vi "Read Write Unit Abbreviations.vi"(0 "Recommended In":T1(array[cluster]), 2 "ServerPath":path, 11 "Error In":errorcluster) -> (4 "Recommended Out":T1(array[cluster]), 8 "[Unit Abbr.s]":string[](array[string]), 10 "[Units]":string[](array[string]), 15 "Error Out":errorcluster)   [LabVIEW 2013]
uses:
  <vilib>/Utility/config.llb/Write Key (String).vi
  <vilib>/Utility/config.llb/Read Key (String).vi
  <vilib>/Utility/config.llb/NI_LVConfig.lvlib
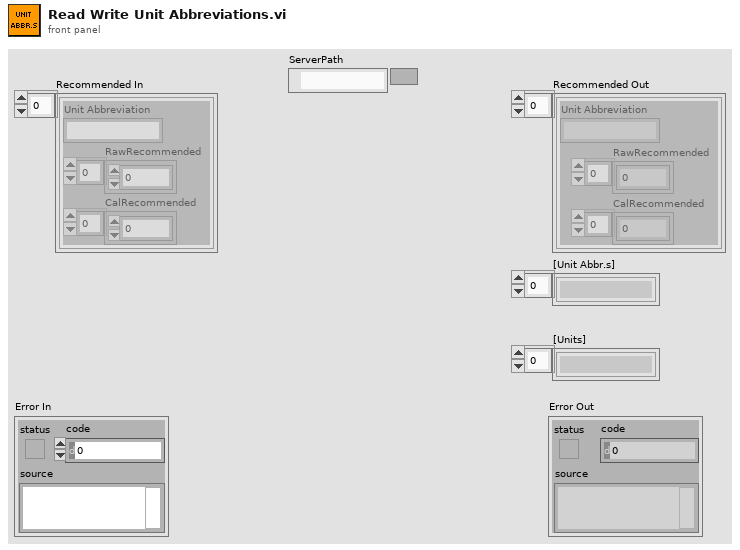
[diagram p1: front panel]
types:
  T1 = cluster{"Unit Abbreviation":string, "RawRecommended":dbl[], "CalRecommended":dbl[]}[]
  T2 = typedef "NI_LVConfig.lvlib/Config Data RefNum.ctl" = refnum<k1>
  T3 = cluster{"Unit Abbreviation":string, "RawRecommended":dbl[], "CalRecommended":dbl[]}
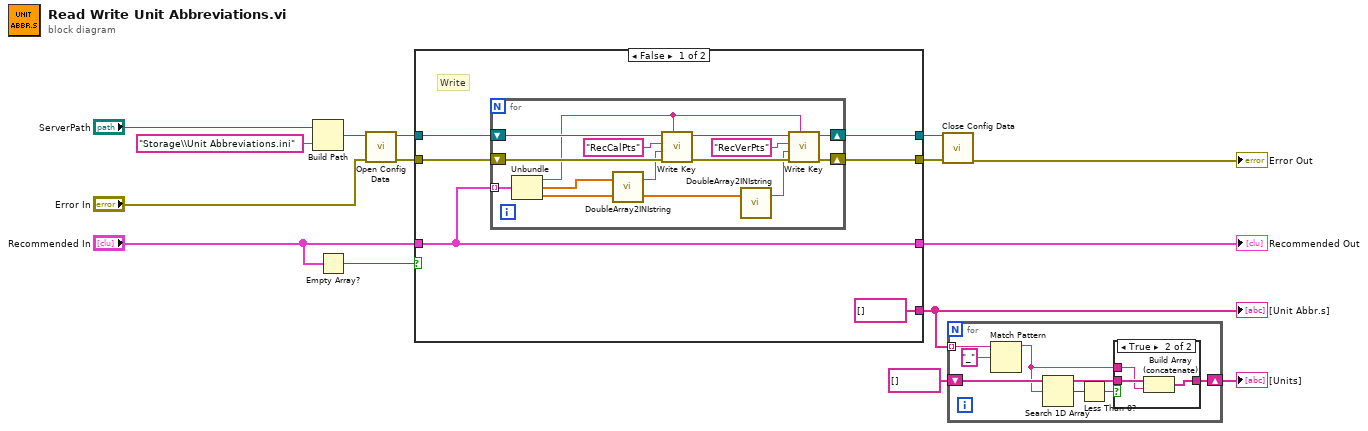
[diagram p0: block diagram]
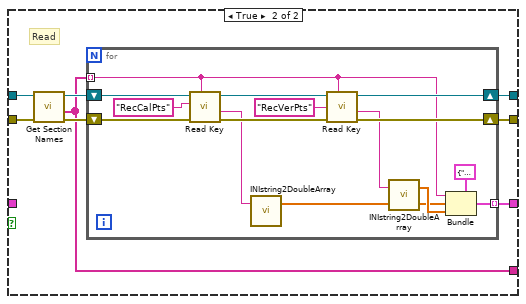
[diagram p3: hidden frame]
diagram:
  n1 = Build Path(base path="ServerPath", name or relative path="Storage\\Unit Abbreviations.ini") -> (appended path=w11:path)
  n2 = Empty Array?(array="Recommended In") -> (empty?=w13:bool)
  n3 = call <vilib>:"Open Config Data.vi"("error in (no error)"="Error In", "configuration file path"=w11) -> ("error out"=w8:errorcluster, "refnum"=w9:T2)  [unwired: 7 in, 1 out]
  n4 = case shown="False" w13 {
    tunnel: "Recommended In" -> [w17 _]
    tunnel: w9 -> [w21 w43]
    tunnel: w8 -> [w20 w42]
    tunnel: [w19 w39] -> w7
    tunnel: [w18 w38] -> w6
    tunnel: [w17 w37] -> w4
    tunnel: [string[] [] ("section names") w36] -> w3
    frame False {
      # "Write"
      n5 = for {
        shift-right: [w29] -> w19
        shift-left: w21 -> [w35]
        shift-right: [w30] -> w18
        shift-left: w20 -> [w34]
        tunnel: w17 -> [w33] mode=indexing
        n6 = Unbundle(w33) -> ("Unit Abbreviation"=w28:string, "RawRecommended"=w25:dbl[], "CalRecommended"=w24:dbl[])
        n7 = call "DoubleArray2INIstring.vi"("Array"=w25) -> ("String"=w22:string)  [unwired: 6 in]
        n8 = call-poly <vilib>:"Write Key.vi"("section"=w28, "error in (no error)"=w34, "value"=w22, "key"="RecCalPts", "refnum"=w35) -> ("error out"=w31:errorcluster, "refnum out"=w32:T2)  [unwired: 4 in, 1 out]
        n9 = call "DoubleArray2INIstring.vi"("Array"=w24) -> ("String"=w23:string)  [unwired: 6 in]
        n10 = call-poly <vilib>:"Write Key.vi"("section"=w28, "error in (no error)"=w31, "value"=w23, "key"="RecVerPts", "refnum"=w32) -> ("error out"=w30:errorcluster, "refnum out"=w29:T2)  [unwired: 4 in, 1 out]
      }
    }
    frame True {
      # "Read"
      n11 = call <vilib>:"Get Section Names.vi"("error in (no error)"=w42, "refnum"=w43) -> ("error out"=w40:errorcluster, "section names"=w36:string[], "refnum out"=w41:T2)  [unwired: 7 in]
      n12 = for {
        shift-right: [w56] -> w39
        shift-left: w41 -> [w58]
        shift-right: [w55] -> w38
        shift-left: w40 -> [w53]
        tunnel: w36 -> [w47] mode=indexing
        tunnel: [w44] -> w37 mode=indexing
        n13 = call-poly <vilib>:"Read Key.vi"("section"=w47, "error in (no error)"=w53, "key"="RecCalPts", "refnum"=w58) -> ("error out"=w54:errorcluster, "value"=w50:string, "refnum out"=w57:T2)  [unwired: 4 in, 1 out]
        n14 = call "INIstring2DoubleArray.vi"("String"=w50) -> ("Array"=w45:dbl[])  [unwired: 6 in]
        n15 = call-poly <vilib>:"Read Key.vi"("section"=w47, "error in (no error)"=w54, "key"="RecVerPts", "refnum"=w57) -> ("error out"=w55:errorcluster, "value"=w49:string, "refnum out"=w56:T2)  [unwired: 4 in, 1 out]
        n16 = call "INIstring2DoubleArray.vi"("String"=w49) -> ("Array"=w46:dbl[])  [unwired: 6 in]
        n17 = Bundle(cluster=T3 {"Unit Abbreviation"="", "RawRecommended"=[], "CalRecommended"=[]}, "Unit Abbreviation"=w47, "RawRecommended"=w45, "CalRecommended"=w46) -> (w44:T3)
      }
    }
  }
  "Recommended Out" <- w4
  "[Unit Abbr.s]" <- w3
  n18 = call <vilib>:"Close Config Data.vi"("error in (no error)"=w6, "refnum"=w7) -> ("error out"=→"Error Out":errorcluster)  [unwired: 8 in, 1 out]
  n19 = for {
    tunnel: w3 -> [w65] mode=indexing
    shift-right: [w59] -> w1
    shift-left: string[] [] -> [w62]
    n20 = Match Pattern(string=w65, regular expression="_") -> (before substring=w61:string)  [unwired: 1 in, 3 out]
    n21 = Search 1D Array(1D array=w62, element=w61) -> (index of element=w63:i32)  [unwired: 1 in]
    n22 = Less Than 0?(x=w63) -> (x < 0?=w60:bool)
    n23 = case shown="True" w60 {
      tunnel: w62 -> [w66 w69]
      tunnel: w61 -> [_ w68]
      tunnel: [w66 w67] -> w59
      frame False {
      }
      frame True {
        n24 = Build Array (concatenate)(w69, w68) -> (w67:string[])
      }
    }
  }
  "[Units]" <- w1
